vi "ShooterPowerMath.vi"(1 "DistanceToTarget":dbl) -> (0 "ShooterPower":dbl)   [LabVIEW 2016]
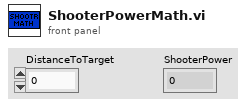
[diagram p1: front panel]
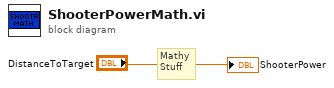
[diagram p0: block diagram]
diagram:
  # "Mathy\nStuff"
  "ShooterPower" <- "DistanceToTarget"
